vi "Get Application Name.vi"() -> (3 "Application":string)   [LabVIEW 2023, in "Logger.lvclass"]
uses:
  Logger.lvclass
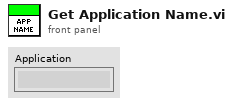
[diagram p1: front panel]
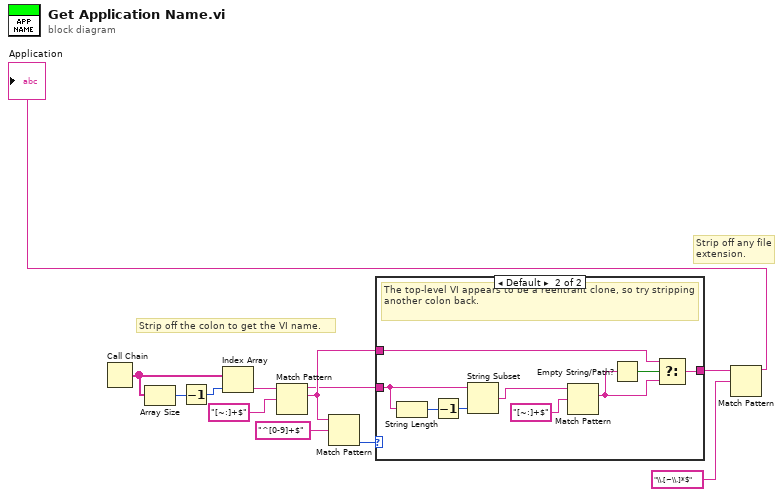
[diagram p0: block diagram]
diagram:
  # "Strip off any file extension."
  # "Strip off the colon to get the VI name."
  n1 = Call Chain() -> (call chain=w3:string[])
  n2 = Array Size(array=w3) -> (size(s)=w2:i32)
  n3 = Decrement(x=w2) -> (x-1=w1:i32)
  n4 = Index Array(array=w3, index=w1) -> (element=w11:string)
  n5 = Match Pattern(string=w11, regular expression="[~:]+$") -> (before substring=w8:string, match substring=w9:string)  [unwired: 1 in, 2 out]
  n6 = Match Pattern(string=w9, regular expression="^[0-9]+$") -> (offset past match=w7:i32)  [unwired: 1 in, 3 out]
  n7 = case shown="Default" w7 {
    tunnel: w8 -> [_ w21]
    tunnel: w9 -> [w13 w14]
    tunnel: [w13 w15] -> w10
    frame -1 {
    }
    frame Default {
      # "The top-level VI appears to be a reentrant clone, so try stripping another colon back."
      n8 = String Length(string=w21) -> (length=w20:i32)
      n9 = Decrement(x=w20) -> (x-1=w19:i32)
      n10 = String Subset(string=w21, length (rest)=w19) -> (substring=w18:string)  [unwired: 1 in]
      n11 = Match Pattern(string=w18, regular expression="[~:]+$") -> (match substring=w16:string)  [unwired: 1 in, 3 out]
      n12 = Empty String/Path?(string/path=w16) -> (empty?=w17:bool)
      n13 = Select(t=w14, s=w17, f=w16) -> (s? t:f=w15:string)
    }
  }
  n14 = Match Pattern(string=w10, regular expression="\\.[~\\.]*$") -> (before substring=→"Application":string)  [unwired: 1 in, 3 out]
